vi "Integrate channel in file.vi"(4 "Buffer size":i64=100000, 6 "Offset duration":dbl=0.0095, 7 "group name in":string="Untitled", 8 "Error In":errorcluster, 10 "Integration settings":T1={"Channel"="", "Output name"="", "Factor"=1.0, "Start time"=nan, "Duration"=nan, "Fix drift"=FALSE} {"Duration" format="%#_6ps"; "Start time" format="%#_6ps"}, 11 "File Path Control":path) -> (0 "Error Out":errorcluster, 2 "Min max":cluster{"Max":dbl, "Min":dbl}, 3 "File Path out":path)   [LabVIEW 2024]
uses:
  <vilib>/Waveform/WDTOps.llb/WDT Number of Waveform Samples DBL.vi
  Utilities/Controls/Integrate channel.ctl
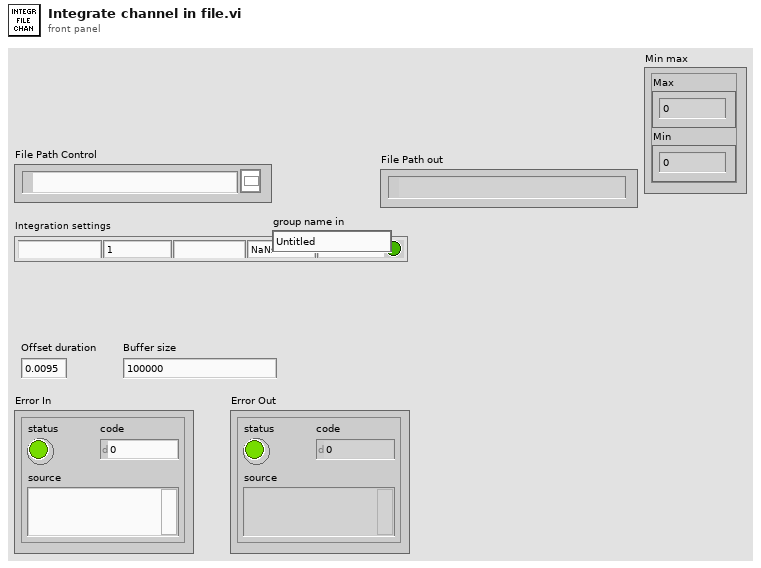
[diagram p1: front panel]
types:
  T1 = typedef "Integrate channel.ctl" = cluster{"Channel":string, "Output name":string, "Factor":dbl, "Start time":dbl, "Duration":dbl, "Fix drift":bool}
  T2 = enum16{"open", "open or create", "create or replace", "create", "open (read-only)"}
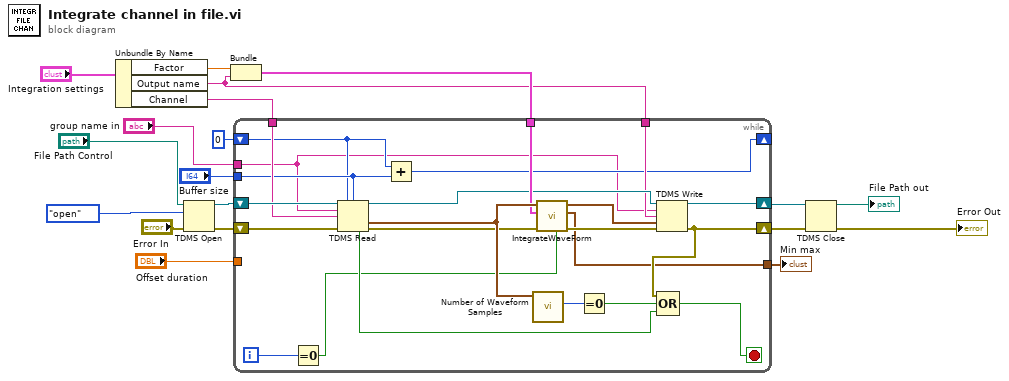
[diagram p0: block diagram]
diagram:
  n1 = Unbundle By Name("Integration settings") -> ("Factor"=w13:dbl, "Output name"=w11:string, "Channel"=w14:string)
  n2 = TDMS Open(8:"Error In", 10:T2."open" ("operation (0:open)"), 11:"File Path Control") -> (0:w10:errorcluster, 3:w16:refnum<k34>)  [unwired: 4 in]
  n3 = Bundle("Factor"=w13, "Output name"=w11) -> (w12:cluster{"Factor":dbl, "Output name":string})  [unwired: 1 in]
  n4 = while {
    tunnel: w14 -> [w40]
    tunnel: w12 -> [w38]
    tunnel: w11 -> [w36]
    shift-right: [w28] -> w9
    shift-left: w10 -> [w31]
    shift-right: [w29] -> w7
    shift-left: w16 -> [w42]
    tunnel: "Buffer size" -> [w26]
    shift-right: [w25] -> _
    shift-left: i64 0 -> [w24]
    tunnel: "Offset duration" -> [_]
    tunnel: [w21] -> w2
    tunnel: "group name in" -> [w20]
    i -> [w23]
    stop <- w30 stop-if-true
    n5 = Equal To 0?(x=w23) -> (x = 0?=w22:bool)
    n6 = TDMS Read(0:w42, 1:w24, 2:w26, 5:w20, 7:w40, 11:w31) -> (4:w37:refnum<k34>, 10:w39:waveform(dbl), 14:w27:bool, 15:w34:errorcluster)  [unwired: 2 in, 2 out]
    n7 = Add(x=w24, y=w26) -> (x+y=w25:i64)
    n8 = call-poly <vilib>:"Number of Waveform Samples.vi"("waveform in"=w39) -> ("number of samples"=w41:i32)  [unwired: 8 in, 2 out]
    n9 = call "IntegrateWaveForm.vi"("First chunk?"=w22, "error in (no error)"=w34, "Integrate settings"=w38, "Waveform"=w39) -> ("error out"=w33:errorcluster, "Min max"=w21:cluster{"Max":dbl, "Min":dbl}, "Integrated Waveform"=w35:waveform(dbl))  [unwired: 5 in]
    n10 = Equal To 0?(x=w41) -> (x = 0?=w32:bool)
    n11 = TDMS Write(0:w37, 5:w20, 7:w36, 9:w35, 11:w33) -> (4:w29:refnum<k34>, 15:w28:errorcluster)  [unwired: 1 in, 2 out]
    n12 = Compound Arithmetic op=OR(w28, w32, w27) -> (w30:bool)
  }
  "Min max" <- w2
  n13 = TDMS Close(8:w9, 11:w7) -> (0:→"Error Out":errorcluster, 3:→"File Path out":path)
